vi "Write Multiple Sections.vi"(7 "error in (no error)":errorcluster, 8 "Section Cluster":variant, 10 "JSON Sections":string="{}") -> (0 "error out":errorcluster, 3 "<JSON>":string caption="<JSON>Sections")   [LabVIEW 2021, in "json.facade.lvlib"]
doc: "Merges a Cluster of Section Clusters (subclusters) into JSON Object. A \"Section Cluster\" is defined in analogy to the OpenG Variant Config Library \"Section Cluster\" functions, using a JSON Object, with subObjects representing \"Sections\", instead of INI format.\n\nMerging means that each element of the Section Cluster is inserted into the JSON \"Section\" (Object Item), using the data name of the cluster element. If a Path to the Section is not specified then the data name of the cluster is used. The Section is created if it does not exist.\n\nFor example, Merging the Cluster \"Settings\" with elements A=123 and B=\"test\" into {\"C\":2,\"Settings\":{\"A\"=6,\"D\":9}} would result in:\n{\"C\":2,\"Settings\":{\"A\"=123,\"D\":9,\"B\":\"test\"}}\n\nNote that this merging is not recursive into subClusters."
uses:
  json.facade.lvlib
  jsontext/JSONtext.lvlib
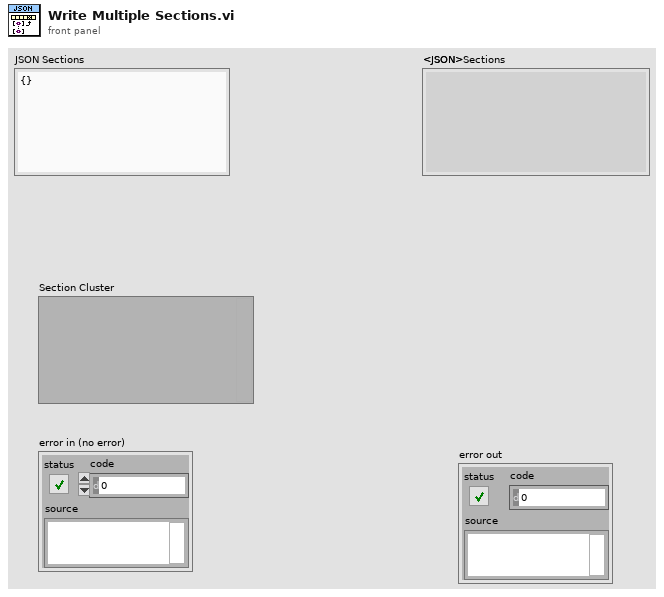
[diagram p1: front panel]
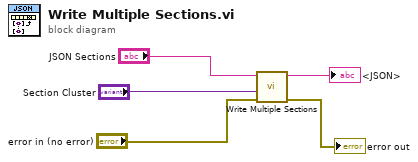
[diagram p0: block diagram]
diagram:
  n1 = call "Write Multiple Sections.vi"("error in (no error)"="error in (no error)", "Section Cluster"="Section Cluster", "JSON Sections"="JSON Sections") -> ("error out"=→"error out":errorcluster, "<JSON>"=→"<JSON>":string)  [unwired: 6 in]
